vi "Toggle Burner.vi"(4 "Timer in":refnum<queue>, 6 "Vesta in":refnum<queue>, 8 "error in (no error)":errorcluster, 11 "Data Cluster In":T1 {"VestaTemperature"."Water Heater Temp (°F)" min=32 max=203}) -> (0 "error out":errorcluster, 3 "Data Cluster out":T1 {"VestaTemperature"."Water Heater Temp (°F)" min=32 max=203})   [LabVIEW 2023]
uses:
  Message Queue/Message Queue.lvlib
  Message Queue/Enqueue Message (Single).vi
  Message Queue/Message Cluster.ctl
  Drivers/Resideo Gas Valve/Type Definitions/Vesta Info.ctl
  controls/Burner Duty Cycle.ctl
  Drivers/Resideo Gas Valve/Type Definitions/Temperature Control.ctl
  controls/UI Data.ctl
  controls/Timer Application Cluster.ctl
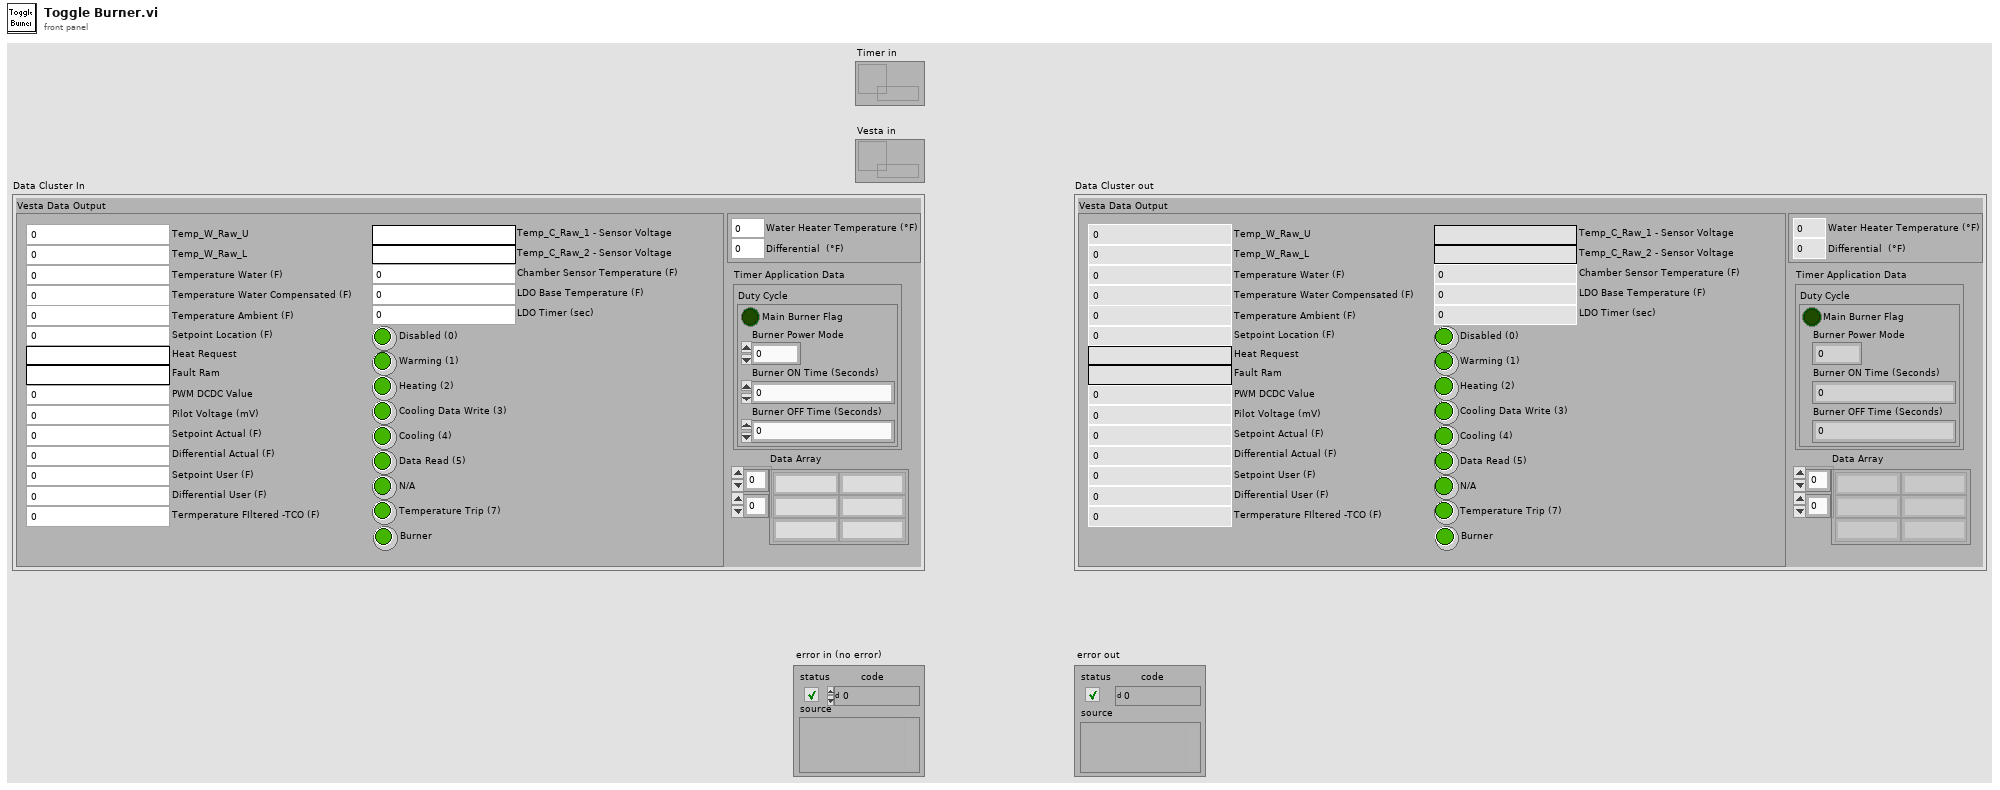
[diagram p1: front panel]
types:
  T1 = typedef "UI Data.ctl" = cluster{"Vesta Data Output":T2, "VestaTemperature":T3, "Timer Application Data":T4, "Data Array":string[][]}
  T2 = typedef "Vesta Info.ctl" = cluster{"Temp_W_Raw_U":u16, "Temp_W_Raw_L":u16, "Temperature Water (F)":dbl, "Temperature Water Compensated (F)":dbl, "Temperature Ambient (F)":dbl, "Setpoint Location (F)":dbl, "Heat Request":string, "Fault Ram":string, "PWM DCDC Value":u16, "Pilot Voltage (mV)":dbl, "Setpoint Actual (F)":dbl, "Differential Actual (F)":dbl, "Setpoint User (F)":dbl, "Differential User (F)":dbl, "Termperature FIltered -TCO (F)":dbl, "Temp_C_Raw_1 - Sensor Voltage":string, "Temp_C_Raw_2 - Sensor Voltage":string, "Chamber Sensor Temperature (F)":dbl, "LDO Base Temperature (F)":dbl, "LDO Timer (sec)":i16, "Disabled (0)":bool, "Warming (1)":bool, "Heating (2)":bool, "Cooling Data Write (3)":bool, "Cooling (4)":bool, "Data Read (5)":bool, "N/A":bool, "Temperature Trip (7)":bool, "Burner":bool}
  T3 = typedef "Temperature Control.ctl" = cluster{"Water Heater Temp (°F)":u16, "Differential  (°F)":dbl}
  T4 = typedef "Timer Application Cluster.ctl" = cluster{"Duty Cycle":T5}
  T5 = typedef "Burner Duty Cycle.ctl" = cluster{"Burner ON Time (Seconds)":dbl, "Burner OFF Time (Seconds)":dbl, "Main Burner Flag":bool, "Burner Power Mode":u8}
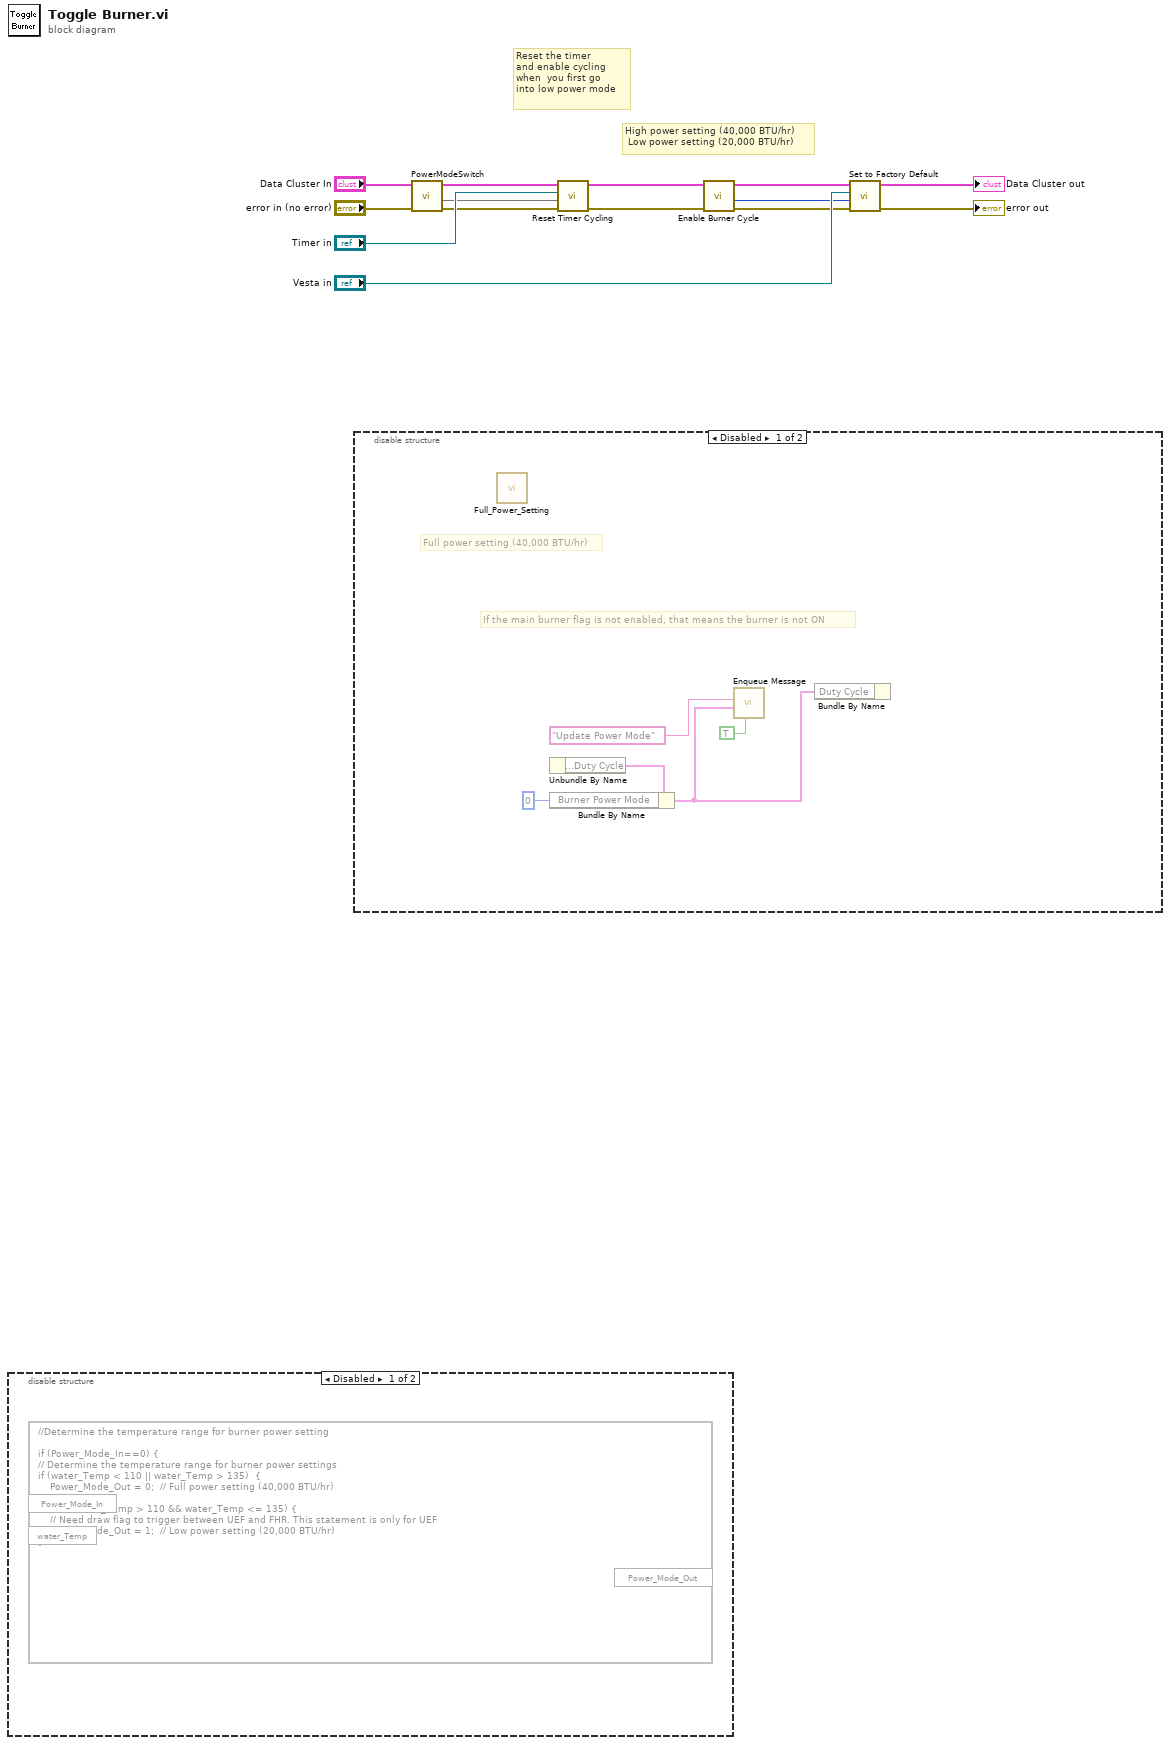
[diagram p0: block diagram]
diagram:
  # "High power setting (40,000 BTU/hr)\n Low power setting (20,000 BTU/hr)"
  # "Reset the timer\nand enable cycling\nwhen  you first go\ninto low power mode"
  n1 = disable-structure shown="Disabled" {
    frame Disabled {
      n2 = formula code="//Determine the temperature range for burner power setting\n\nif (Power_Mode_In==0) {\n// Determine the temperature range for burner power settings\nif (water_Temp < 110 || water_Temp > 135)  {\n    Power_Mode_Out = 0;  // Full power setting (40,000 BTU/hr)\n} \nelse if (water_Temp > 110 && water_Temp <= 135) {\n    // Need draw flag to trigger between UEF and FHR. This statement is only for UEF\n    Power_Mode_Out = 1;  // Low power setting (20,000 BTU/hr)\n}"() -> ()  [unwired: 2 in, 1 out]
    }
    frame Enabled {
    }
  }
  n3 = disable-structure shown="Disabled" {
    frame Disabled {
      # "If the main burner flag is not enabled, that means the burner is not ON"
      # "Full power setting (40,000 BTU/hr)"
      n4 = call "Full_Power_Setting.vi"() -> ()  [unwired: 10 in, 2 out]
      n5 = Unbundle By Name() -> ("Timer Application Data.Duty Cycle"=w18:T5)  [unwired: 1 in]
      n6 = Bundle By Name(cluster=w18, "Burner Power Mode"=u8 0 ("Timer Application Data.Duty Cycle.Burner Power Mode")) -> (w19:T5)
      n7 = call-poly "Enqueue Message.vi"("Priority Message? (F)"=TRUE, "Message Data"=w19, "Message"="Update Power Mode") -> ()  [unwired: 7 in, 2 out]
      n8 = Bundle By Name("Duty Cycle"=w19) -> ()  [unwired: 1 in, 1 out]
    }
    frame Enabled {
    }
  }
  n9 = call "PowerModeSwitch.vi"("error in (no error)"="error in (no error)", "Data Cluster In"="Data Cluster In") -> ("error out"=w8:errorcluster, 1:w5, "Data Cluster out"=w4:T1)  [unwired: 5 in, 2 out]
  n10 = call "Reset Timer Cycling.vi"("error in (no error)"=w8, "Send_Timer_Message"=w5, 10:"Timer in", "Data Cluster In"=w4) -> ("error out"=w7:errorcluster, "Data Cluster Output"=w6:T1)  [unwired: 6 in]
  n11 = call "Enable Burner Cycle.vi"("error in (no error)"=w7, "Data Cluster In"=w6) -> ("error out"=w3:errorcluster, "Send_Vesta_Message"=w1:u8, "Data Cluster Output"=w2:T1)  [unwired: 7 in]
  n12 = call "Set to Factory Default.vi"("error in (no error)"=w3, "Send_Vesta_Message"=w1, "Vesta in"="Vesta in", "Data Cluster In"=w2) -> ("error out"=→"error out":errorcluster, "Data Cluster Out"=→"Data Cluster out":T1)  [unwired: 6 in]
